vi "getCenter.vi"(8 "error in (no error)":errorcluster, 11 "GObject in":refnum<class "GObject.lvclass">) -> (0 "error out":errorcluster, 2 "center":T1, 3 "GObject out":refnum<class "GObject.lvclass">)   [LabVIEW 2023, in "TLC_Scripto.lvlib" / "GObject.lvclass"]
uses:
  GObject.lvclass
  Ctrls/point.ctl
  TLC_Scripto.lvlib
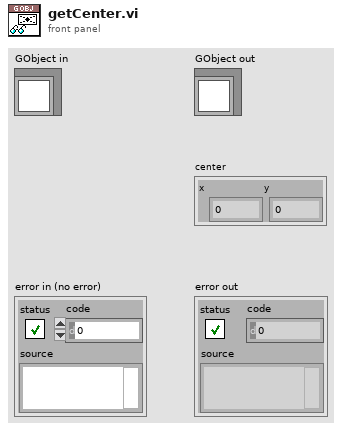
[diagram p1: front panel]
types:
  T1 = typedef "TLC_Scripto.lvlib/point.ctl" = cluster{"x":i32, "y":i32}
  T2 = typedef "TLC_Scripto.lvlib/rectangle.ctl" = cluster{"left":i32, "top":i32, "right":i32, "bottom":i32}
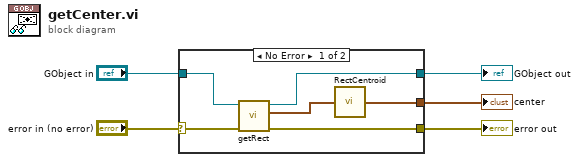
[diagram p0: block diagram]
diagram:
  n1 = case shown="No Error" "error in (no error)" {
    selector: "error in (no error)" -> [w11 w13]
    tunnel: [w7 w13] -> w4
    tunnel: [w9 w12] -> w2
    tunnel: "GObject in" -> [w8 w12]
    tunnel: [w6 _] -> w1
    frame No Error {
      n2 = call-dynamic "getRect.vi"("error in (no error)"=w11, "GObject in"=w8) -> ("error out"=w7:errorcluster, "rectangle"=w10:T2, "GObject out"=w9:refnum<class "GObject.lvclass">)  [unwired: 7 in]
      n3 = call <vilib>:"RectCentroid.vi"("rect"=w10) -> ("point"=w6:cluster{"x":i16, "y":i16})
    }
    frame Error {
    }
  }
  "error out" <- w4
  "GObject out" <- w2
  "center" <- w1
